vi "Decode TextString.vi"(11 "Length-Prefixed Field":u8[](array[numeric]) format="%08x") -> (2 "Text String":string, 3 "Remaining Packets":u8[](array[numeric]) format="%08b", 5 "restricted code":bool)   [LabVIEW 2013, in "MQTT_Control_Packets.lvlib" / "ControlPacket.lvclass"]
uses:
  ControlPacket.lvclass
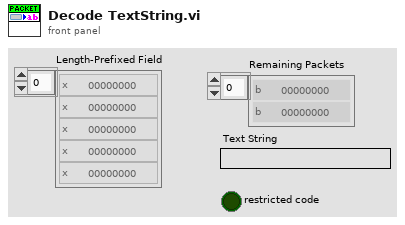
[diagram p1: front panel]
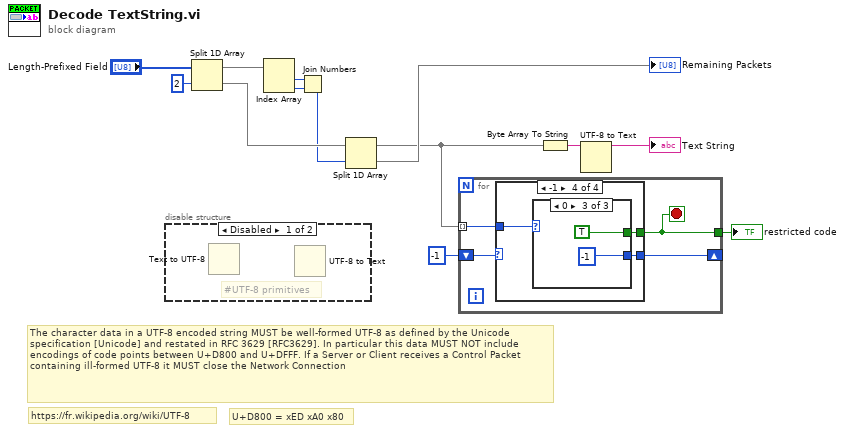
[diagram p0: block diagram]
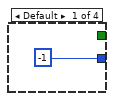
[diagram p2: hidden frame]
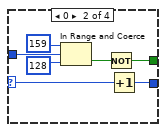
[diagram p3: hidden frame]
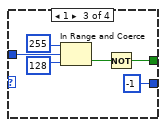
[diagram p4: hidden frame]
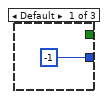
[diagram p5: hidden frame]
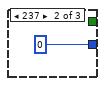
[diagram p6: hidden frame]
diagram:
  # "U+D800 = xED xA0 x80"
  # "https://fr.wikipedia.org/wiki/UTF-8"
  # "The character data in a UTF-8 encoded string MUST be well-formed UTF-8 as defined by the Unicode specification [Unicode] and restated in RFC 3629 [RFC3629]. In particular this data MUST NOT include encodings of code points between U+D800 and U+DFFF. If a Server or Client receives a Control Packet containing ill-formed UTF-8 it MUST close the Network Connection"
  n1 = disable-structure shown="Disabled" {
    frame Disabled {
      # "#UTF-8 primitives"
      n2 = Text to UTF-8() -> ()  [unwired: 2 in, 2 out]
      n3 = UTF-8 to Text() -> ()  [unwired: 2 in, 2 out]
    }
    frame Enabled {
    }
  }
  n4 = Split 1D Array(array="Length-Prefixed Field", index=2) -> (first subarray=w12:u8[], second subarray=w11:u8[])
  n5 = Index Array(array=w12) -> (element #1=w9:u8, element #2=w10:u8)  [unwired: 2 in]
  n6 = Join Numbers(hi=w9, lo=w10) -> ((hi.lo)=w8:u16)
  n7 = Split 1D Array(array=w11, index=w8) -> (first subarray=w4:u8[], second subarray=→"Remaining Packets":u8[])
  n8 = for {
    tunnel: w4 -> [w17] mode=indexing
    shift-right: [w16] -> _
    shift-left: -1 -> [w15]
    tunnel: [w14] -> w3
    stop <- w14 stop-if-true
    n9 = case shown="-1" w15 {
      selector: w15 -> [_ w24 _ _]
      tunnel: w17 -> [_ w19 w26 w34]
      tunnel: [-1 w25 -1 w33] -> w16
      tunnel: [_ w20 w28 w32] -> w14
      frame Default {
      }
      frame 0 {
        n10 = In Range and Coerce(upper limit=u8 159 ("Byte"), x=w19, lower limit=u8 128 ("Byte")) -> (In Range?=w21:bool)  [unwired: 1 out]
        n11 = Not(x=w21) -> (.not. x?=w20:bool)
        n12 = Increment(x=w24) -> (x+1=w25:i32)
      }
      frame 1 {
        n13 = In Range and Coerce(upper limit=u8 255 ("Byte"), x=w26, lower limit=u8 128 ("Byte")) -> (In Range?=w29:bool)  [unwired: 1 out]
        n14 = Not(x=w29) -> (.not. x?=w28:bool)
      }
      frame -1 {
        n15 = case shown="0" w34 {
          tunnel: [-1 0 -1] -> w33
          tunnel: [_ _ TRUE] -> w32
          frame Default {
          }
          frame 237 {
          }
          frame 0 {
          }
        }
      }
    }
  }
  "restricted code" <- w3
  n16 = Byte Array To String(unsigned byte array=w4) -> (string=w2:string)
  n17 = UTF-8 to Text(11:w2) -> (3:→"Text String":string)  [unwired: 1 in, 1 out]
